vi "cartoon.vi"(4 "Jackie Chan":T1, 6 "Ben10":T3, 8 "Spiderman":T2, 10 "Dragon Booster":bool, 11 "Error in":errorcluster) -> (15 "Error out":errorcluster)   [LabVIEW 2020]
uses:
  Custom controls/Cartoon2.ctl
  Custom controls/Cartoon3.ctl
  Custom controls/Cartoon4.ctl
panel:
  in  "Next":bool
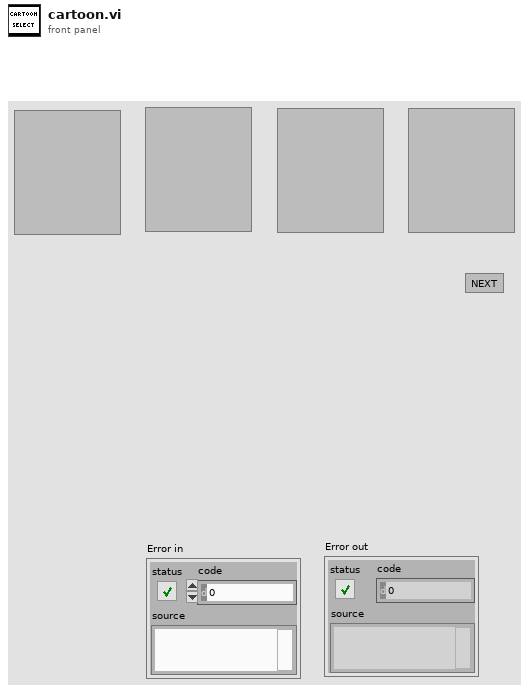
[diagram p1: front panel]
types:
  T1 = typedef "Cartoon4.ctl" = bool
  T2 = typedef "Cartoon3.ctl" = bool
  T3 = typedef "Cartoon2.ctl" = bool
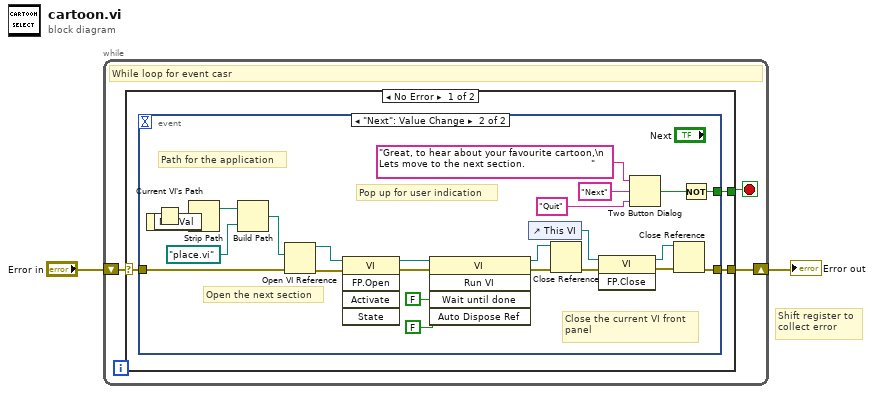
[diagram p0: block diagram]
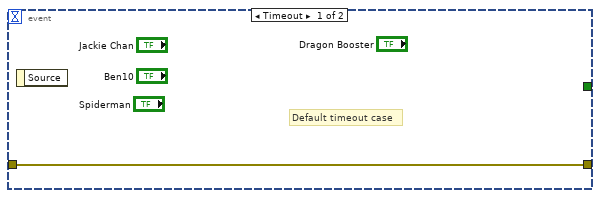
[diagram p2: hidden frame]
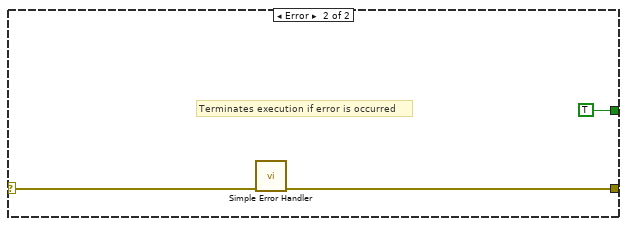
[diagram p3: hidden frame]
diagram:
  # "Shift register to \ncollect error"
  n1 = while {
    shift-right: [w4] -> w1
    shift-left: "Error in" -> [w5]
    stop <- w3 stop-if-true
    # "While loop for event casr"
    n2 = case shown="No Error" w5 {
      selector: w5 -> [w8 w35]
      tunnel: [w7 w34] -> w4
      tunnel: [w6 TRUE] -> w3
      frame No Error {
        n3 = event shown="[1] \"Next\": Value Change" {
          selector: _ -> [_ _]
          dyn-events: _ -> [_ _]
          timeout: _ -> [_ _]
          tunnel: w8 -> [w9 w10]
          tunnel: [w9 w21] -> w7
          tunnel: [_ w28] -> w6
          event Timeout {
            # "Default timeout case"
            n4 = event-data() -> ()  [unwired: 1 in, 1 out]
          }
          event "Next": Value Change {
            # "Path for the application"
            # "Pop up for user indication"
            # "Open the next section"
            # "Close the current VI front\npanel"
            n5 = event-data() -> ()  [unwired: 1 in, 1 out]
            n6 = Current VI's Path() -> (path=w19:path)
            n7 = Strip Path(path=w19) -> (stripped path=w18:path)  [unwired: 1 out]
            n8 = Build Path(base path=w18, name or relative path=path "place.vi") -> (appended path=w17:path)
            n9 = Open VI Reference(vi path=w17, error in (no error)=w10) -> (vi reference=w27:refnum<vi>, error out=w26:errorcluster)  [unwired: 4 in]
            n10 = invoke class="VI" method="FP.Open"(reference=w27, error in=w26) -> (reference out=w24:refnum<vi>, error out=w25:errorcluster)  [unwired: 3 in, 3 out]
            n11 = invoke class="VI" method="Run VI"(reference=w24, error in=w25, "Wait until done"=FALSE ("Wait Until Done"), "Auto Dispose Ref"=FALSE ("Auto Dispose Reference")) -> (reference out=w12:refnum<vi>, error out=w16:errorcluster)  [unwired: 1 in, 3 out]
            n12 = control-ref of="This VI"() -> (w11:refnum<vi>)
            n13 = Close Reference(reference=w12, error in (no error)=w16) -> (error out=w15:errorcluster)
            n14 = invoke class="VI" method="FP.Close"(reference=w11, error in=w15) -> (reference out=w13:refnum<vi>, error out=w14:errorcluster)  [unwired: 1 in, 1 out]
            n15 = Two Button Dialog(message="Great, to hear about your favourite cartoon,\n Lets move to the next section.                      ", 1:"Quit" ("F button name (\"Cancel\")"), 2:"Next" ("T button name (\"OK\")")) -> (T button?=w29:bool)
            n16 = Close Reference(reference=w13, error in (no error)=w14) -> (error out=w21:errorcluster)
            n17 = Not(x=w29) -> (.not. x?=w28:bool)
          }
        }
      }
      frame Error {
        # "Terminates execution if error is occurred"
        n18 = call <vilib>:"Simple Error Handler.vi"("error in (no error)"=w35) -> ("error out"=w34:errorcluster)  [unwired: 4 in, 4 out]
      }
    }
  }
  "Error out" <- w1
